vi "PH_StatusHandler.panel.vi"(0 "object ref":refnum<vi>, 5 "error in (no error)":errorcluster) -> (19 "error out":errorcluster)   [LabVIEW 2014, in "PH_StatusHandler.lvlib"]
doc: "By this VI a hardware switch can be monitored and switched. \n\nThe indicators \"FALSE\", \"TRUE\" and \"SWITCH STATE\" show the value of the Beckhoff-Tag: blue indicates bad tag status reference problems, darkgreen false and lightgreen true. If everything is working fine, \"FALSE\" and \"SWITCH STATE\" should show the same value, while \"TRUE\" has the opposite value. The caption of the sensors for \"FALSE\" and \"TRUE\" are taken out of the database. In case of only one or no sensor these GUI elements are not shown at all.\n\nThe oval button switches. It should be in the same state as the \"SWITCH STATE\" indicator. \n\n\"Delete Instance\" disconnects and removes the instance from the PCS.\n\n\nLicense Agreement for this software:\n\nCopyright (C)\nGesellschaft für Schwerionenforschung, GSI\nPlanckstr. 1\n64291 Darmstadt\nGermany\n\nContact: D.Beck@gsi.de \n\nThis program is free software; you can redistribute it and/or modify it under the terms of the GNU General Public License as published by the Free Software Foundation; either version 2 of the license, or (at your option) any later version.\n\nThis program is distributed in the hope that it will be useful, but WITHOUT ANYW ARRANTY; without even the implied warranty of MERCHANTABILITY or FITNESS FOR A PARTICULAR PURPOSE. See the GNU General License for more details (http://www.gnu.org).\n\nGesellschaft für Schwerionenforschung, GSI\nPlanckstr. 1, 64291 Darmstadt, Germany\nFor all questions and ideas contact: M.Richter@gsi.de, H.Brand@gsi.de or D.Beck@gsi.de.\nLast update: 18-DEC-2002"
uses:
  PH_StatusHandler.lvlib
  PH_StatusHandler.GUI element.ctl
  PH_Common/PH_Common.lvlib
  PH_Class/PH_Class.lvlib
panel:
  out "Status":T1
  in  "Delete":bool
  # "PCS"
  # "3.40"
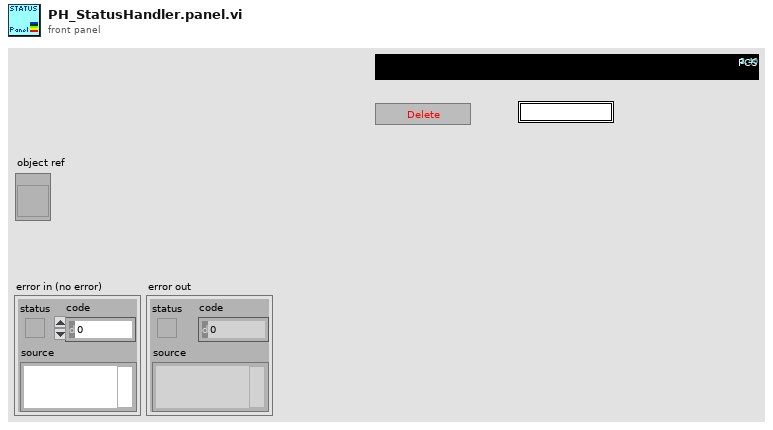
[diagram p1: front panel]
types:
  T1 = typedef "PH_StatusHandler.lvlib/PH_StatusHandler.GUI element.ctl" = u16
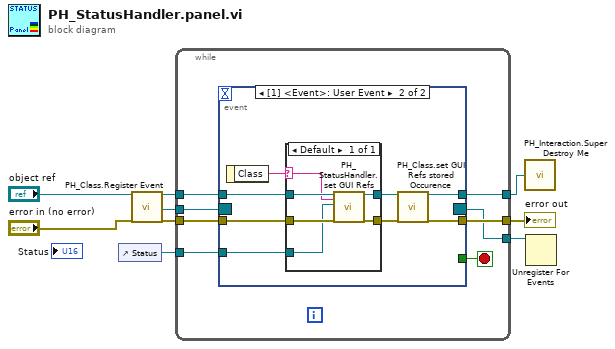
[diagram p0: block diagram]
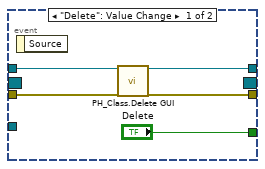
[diagram p2: hidden frame]
diagram:
  n1 = control-ref of="Status"() -> (w1:refnum<vi>)
  n2 = call "PH_Class.Register Event.vi"("i ref in"="object ref", "error in (no error)"="error in (no error)") -> ("i ref out"=w4:refnum<vi>, "Event Registration Refnum"=w3:refnum<event-registration>, "error out"=w5:errorcluster)  [unwired: 15 in]
  n3 = while {
    tunnel: w4 -> [w14]
    tunnel: [w13] -> w9
    tunnel: w5 -> [w16]
    tunnel: [w15] -> w8
    tunnel: w3 -> [w12]
    tunnel: [w11] -> w2
    tunnel: w1 -> [w10]
    stop <- w17 stop-if-true
    n4 = event shown="[1] <Event>: User Event" {
      selector: w12 -> [_ _]
      dyn-events: [_ _] -> w11
      timeout: _ -> [_ _]
      tunnel: ["Delete" _] -> w17
      tunnel: w14 -> [w18 w30]
      tunnel: w16 -> [w19 w29]
      tunnel: [w21 w25] -> w15
      tunnel: [w20 w24] -> w13
      tunnel: w10 -> [_ w27]
      event "Delete": Value Change {
        n5 = event-data() -> ()  [unwired: 1 in, 1 out]
        n6 = call "PH_Class.Delete GUI.vi"("VI in"=w18, "error in (no error)"=w19) -> ("VI out"=w20:refnum<vi>, "error out"=w21:errorcluster)  [unwired: 16 in]
      }
      event User Event {
        n7 = event-data() -> ("Class"=w26:string)  [unwired: 1 in]
        n8 = case shown="Default" w26 {
          selector: w26 -> [w31]
          tunnel: w30 -> [w36]
          tunnel: [w35] -> w23
          tunnel: w29 -> [w34]
          tunnel: [w33] -> w28
          tunnel: w27 -> [w32]
          frame Default {
            n9 = call "PH_StatusHandler.set GUI Refs.vi"("i ref in"=w36, "Class"=w31, "GUI Ref"=w32, "error in (no error)"=w34) -> ("i ref out"=w35:refnum<vi>, "error out"=w33:errorcluster)  [unwired: 14 in]
          }
        }
        n10 = call "PH_Class.set GUI Refs stored Occurence.vi"("i ref in"=w23, "error in (no error)"=w28) -> ("i ref out"=w24:refnum<vi>, "error out"=w25:errorcluster)  [unwired: 16 in]
      }
    }
  }
  "error out" <- w8
  n11 = call "PH_Interaction.Super Destroy Me.vi"("i ref out"=w9) -> ()
  n12 = Unregister For Events(event registration refnum=w2) -> ()  [unwired: 1 in, 1 out]
